vi "ColorSensorRefNum Registry Set.vi"(8 "error in (no error)":errorcluster, 9 "Test Mode Only":bool, 10 "refnum name":string="ColorSensor", 11 "ColorSensorDevRef":T1={"I2CDevRef"={"DevStatus"={"status"=FALSE, "code"=0, "source"=""}, "Device Address"=0, "Handle"=0, "I2C Bus"=enum."Invalid"}} {"I2CDevRef"."Device Address" format="%.0x"}) -> (0 "error out":errorcluster, 3 "ColorSensorDevRef out":T1={"I2CDevRef"={"DevStatus"={"status"=FALSE, "code"=0, "source"=""}, "Device Address"=0, "Handle"=0, "I2C Bus"=enum."Invalid"}} {"I2CDevRef"."Device Address" format="%.0x"})   [LabVIEW 2018, in "ColorSensor.lvlib"]
uses:
  ColorSensor.lvlib
  TypeDef/ColorSensorDevRef.ctl
  <vilib>/Rock Robotics/WPI/I2C/WPI_I2CDevRef.ctl
  <vilib>/Rock Robotics/SystemInterfaces/i2clib/i2c_bus.ctl
  <vilib>/Rock Robotics/WPI/Utilities/Refnum Registry Operation.ctl
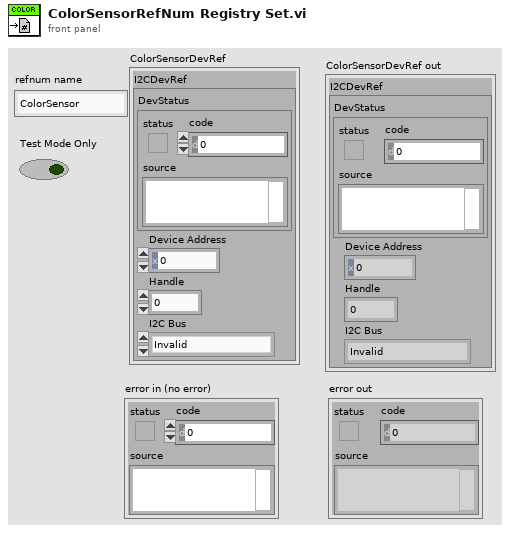
[diagram p1: front panel]
types:
  T1 = typedef "ColorSensor.lvlib/ColorSensorDevRef.ctl" = cluster{"I2CDevRef":T2}
  T2 = typedef "WPI_I2CDevRef.ctl" = cluster{"DevStatus":errorcluster, "Device Address":u8, "Handle":i32, "I2C Bus":T3}
  T3 = typedef "i2c_bus.ctl" = enum16{"I2C On-Board", "I2C MXP", "Invalid"}
  T4 = typedef "Refnum Registry Operation.ctl" = enum16{"set", "get", "delete", "get all names", "read name"}
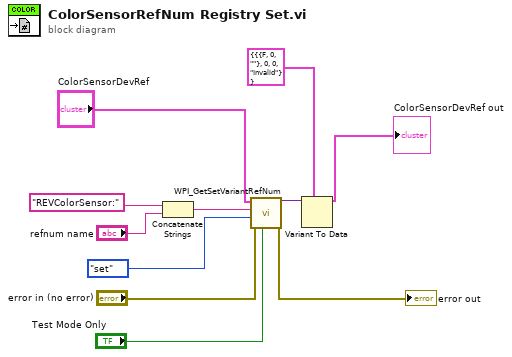
[diagram p0: block diagram]
diagram:
  n1 = Concatenate Strings("REVColorSensor:", "refnum name") -> (w11:string)
  n2 = call <vilib>:"WPI_GetSetVariantRefNum.vi"("Test Mode Only"="Test Mode Only", "error in (no error)"="error in (no error)", "Operation"=Refnum_Registry_Operation."set" ("menu"), "refnum name"=w11, "DevRef"="ColorSensorDevRef") -> ("error out"=→"error out":errorcluster, "DevRef"=w9:variant)  [unwired: 4 in, 1 out]
  n3 = Variant To Data(type=T1 {"I2CDevRef"={"DevStatus"={"status"=FALSE, "code"=0, "source"=""}, "Device Address"=0, "Handle"=0, "I2C Bus"=enum."Invalid"}} ("ColorSensorDevRef"), Variant=w9) -> (data=→"ColorSensorDevRef out":T1)  [unwired: 1 in, 1 out]
